vi "Chart - Buffer Data.vi"(5 "clear first (no:F)":bool, 7 "Time":dbl, 11 "Data":dbl) -> (3 "XY chart data":cluster{"x":dbl, "y":dbl}[](array[cluster]) {"y" format="%.2f"; "x" format="%.2f"})   [LabVIEW 2014]
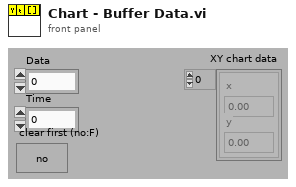
[diagram p1: front panel]
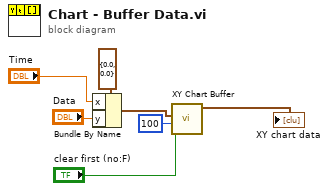
[diagram p0: block diagram]
diagram:
  n1 = Bundle By Name(cluster=cluster{"x":dbl, "y":dbl} {"x"=0.0, "y"=0.0} ("new point"), "x"="Time", "y"="Data") -> (w5:cluster{"x":dbl, "y":dbl})
  n2 = call "XY Chart Buffer.vi"("clear first (no:F)"="clear first (no:F)", "chart length (points)"=100, "new point"=w5) -> ("XY chart data"=→"XY chart data":cluster{"x":dbl, "y":dbl}[])  [unwired: 8 in]
